vi "wait.vi"(0 "HGF_DIMEvent":refnum<class "HGF_DIMEvent.lvclass">, 3 "msTimeout (-1)":i32=-1, 5 "error in (no error)":errorcluster, 9 "ignore previous (F)":bool) -> (14 "dup HGF_DIMEvent":refnum<class "HGF_DIMEvent.lvclass">, 16 "Object":refnum<class>, 17 "timed out":bool, 19 "error out":errorcluster)   [LabVIEW 2012, in "HGF_DIM.lvlib" / "HGF_DIMEvent.lvclass"]
doc: "Use this VI to wait on events.\n\n<b>Hint:</b> This is a shared reentrant VI."
uses:
  HGF_DIMEvent.lvclass
  HGF_DIMEvent.lvclass/HGF_DIMEvent.ctl
  HGF_Auxiliary/Severity.ctl
  HGF_Auxiliary/ErrorCode.ctl
  HGF_BaseClasses/HGF_Event/HGF_Event.lvclass
  HGF_BaseClasses/HGF_Timing/HGF_Timing.lvclass
  HGF_Auxiliary/HGF_Auxiliary.lvlib
  DimLVEvent/LVDimInterface/LVDimInterface.lvlib
  HGF_BaseClasses/HGF_NetworkEvent/HGF_NetworkEvent.lvclass/HGF_NetworkEvent.lvclass
  HGF_BaseClasses/HGF_NetworkVisitor/HGF_NetworkVisitor.lvclass
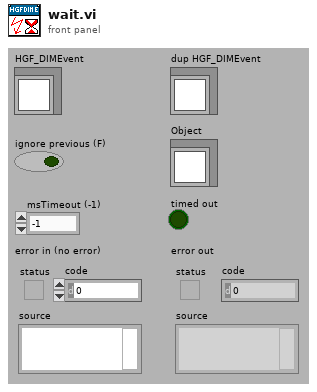
[diagram p1: front panel]
types:
  T1 = typedef "HGF_Auxiliary.lvlib/ErrorCode.ctl" = enum32{"No error", "Function not supported.", "This VI is for friends only.", "Reference object aready exisits.", "Parameter out of range.", "Not a rendezvous.", "Invalid notifier reference.", "Invalid queue reference.", "Self-Test not supported.", "Reset not supported.", "IDN query not supported.", "Error query not supported.", "Incorrect addressee.", "Object already exists.", "No class name specified", "Driver not supported", "Attribute is not writable"}
  T2 = typedef "HGF_Auxiliary.lvlib/Severity.ctl" = enum16{"Info", "Warning", "Fault", "Error", "Fatal"}
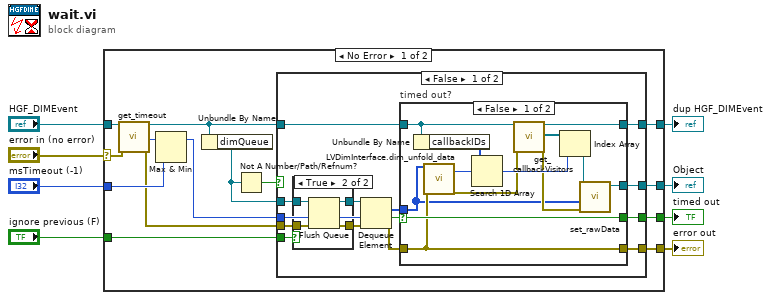
[diagram p0: block diagram]
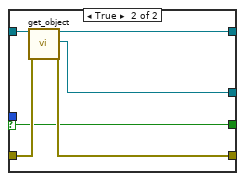
[diagram p2: hidden frame]
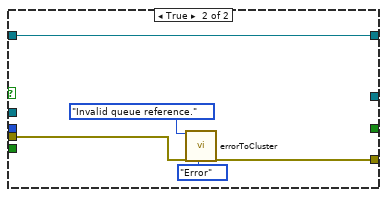
[diagram p4: hidden frame]
diagram:
  n1 = case shown="No Error" "error in (no error)" {
    selector: "error in (no error)" -> [w18 _]
    tunnel: "HGF_DIMEvent" -> [w22 w67]
    tunnel: [w10 w67] -> w4
    tunnel: [w21 _] -> w2
    tunnel: [w20 _] -> w3
    tunnel: [w19 _] -> w1
    tunnel: "msTimeout (-1)" -> [w15 _]
    tunnel: "ignore previous (F)" -> [w13 _]
    frame No Error {
      n2 = call "get_timeout.vi"("HGF_Event.lvclass in"=w22, "error in (no error)"=w18) -> ("HGF_Event.lvclass out"=w9:refnum<class "HGF_DIMEvent.lvclass">, "timeout"=w17:i32, "error out"=w14:errorcluster)  [unwired: 15 out]
      n3 = Max & Min(x=w17, y=w15) -> (max(x,y)=w16:i32)  [unwired: 1 out]
      n4 = Unbundle By Name(w9) -> ("dimQueue"=w11:refnum<queue>)
      n5 = Not A Number/Path/Refnum?(number/path/refnum=w11) -> (NaN/Path/Refnum?=w12:bool)
      n6 = case shown="False" w12 {
        tunnel: [w27 _] -> w21
        tunnel: [w26 _] -> w20
        tunnel: [w23 w66] -> w19
        tunnel: w16 -> [w36 _]
        tunnel: w11 -> [w35 _]
        tunnel: w14 -> [w33 w64]
        tunnel: w13 -> [w31 _]
        tunnel: [w29 w62] -> w10
        tunnel: w9 -> [w30 w62]
        frame False {
          n7 = case shown="True" w31 {
            tunnel: w35 -> [w57 w61]
            tunnel: [w57 w60] -> w34
            tunnel: w33 -> [w56 w59]
            tunnel: [w56 w58] -> w32
            frame False {
            }
            frame True {
              n8 = Flush Queue(queue=w61, error in (no error)=w59) -> (queue out=w60:refnum<queue>, error out=w58:errorcluster)  [unwired: 1 out]
            }
          }
          n9 = Dequeue Element(queue=w34, timeout in ms (-1)=w36, error in (no error)=w32) -> (element=w25:i8[], timed out?=w28:bool, error out=w24:errorcluster)  [unwired: 1 out]
          n10 = case "timed out?" shown="False" w28 {
            selector: w28 -> [w49 w51]
            tunnel: w30 -> [w46 w55]
            tunnel: [w45 w54] -> w29
            tunnel: w24 -> [w40 w53]
            tunnel: [w40 w52] -> w23
            tunnel: [w49 w51] -> w27
            tunnel: [w41 w50] -> w26
            tunnel: w25 -> [w37 _]
            frame False {
              n11 = Unbundle By Name(w46) -> ("callbackIDs"=w48:i32[])
              n12 = call "LVDimInterface.dim_unfold_data.vi"("rawData"=w37, "error in (no error)"=w40) -> ("callBackID"=w47:i32, "error out"=w39:errorcluster)  [unwired: 16 out]
              n13 = Search 1D Array(1D array=w48, element=w47) -> (index of element=w43:i32)  [unwired: 1 out]
              n14 = call "get_callbackVisitors.vi"("HGF_NetworkEvent"=w46, "error in (no error)"=w39) -> ("dup HGF_NetworkEvent"=w45:refnum<class "HGF_DIMEvent.lvclass">, "callbackVisitors"=w44:refnum<class "HGF_NetworkVisitor.lvclass">[], "error out"=w38:errorcluster)  [unwired: 15 out]
              n15 = Index Array(array=w44, index=w43) -> (element=w42:refnum<class "HGF_NetworkVisitor.lvclass">)
              n16 = call "set_rawData.vi"("error in (no error)"=w38, "rawData"=w37, "HGF_NetworkData"=w42) -> ("dup HGF_NetworkData"=w41:refnum<class "HGF_NetworkVisitor.lvclass">)  [unwired: 8 out]
            }
            frame True {
              n17 = call "get_object.vi"("HGF_Timing.lvclass"=w55, "error in (no error)"=w53) -> ("dup HGF_Timing"=w54:refnum<class "HGF_DIMEvent.lvclass">, "object"=w50:refnum<class>, "error out"=w52:errorcluster)  [unwired: 15 out]
            }
          }
        }
        frame True {
          n18 = call "errorToCluster.vi"("error code"=ErrorCode."Invalid queue reference.", "error in (no error)"=w64, "severity (Error)"=Severity."Error") -> ("error out"=w66:errorcluster)  [unwired: 2 in, 14 out]
        }
      }
    }
    frame Error {
    }
  }
  "error out" <- w1
  "dup HGF_DIMEvent" <- w4
  "timed out" <- w2
  "Object" <- w3
